vi "Get Enumerator.vi"(8 "error in (no error)":errorcluster caption="错误输入（无错误）", 11 "ArrayListClass 输入":refnum<class "ArrayListClass.lvclass"> caption="DNL_LabVIEW Object in") -> (0 "error out":errorcluster caption="错误输出", 2 "Enumerator 输出":refnum<class "Enumerator.lvclass">, 3 "ArrayListClass 输出":refnum<class "ArrayListClass.lvclass"> caption="DNL_LabVIEW Object out")   [LabVIEW 2012, in "ArrayListClass.lvclass"]
uses:
  ArrayListClass.lvclass
  Enumerator/Enumerator.lvclass
  ArrayListClass.lvclass/ArrayListClass.ctl
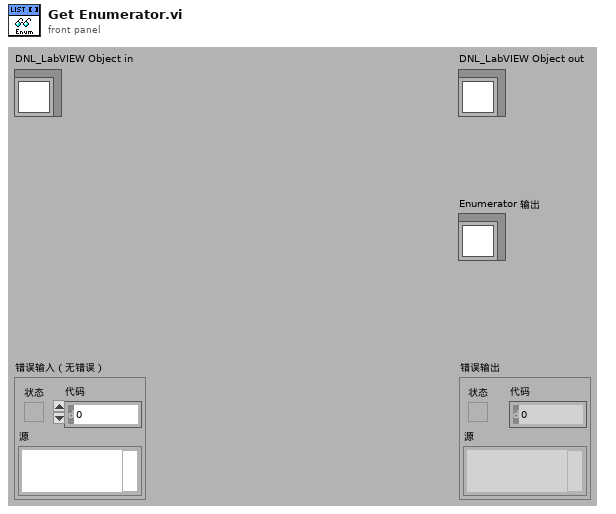
[diagram p1: front panel]
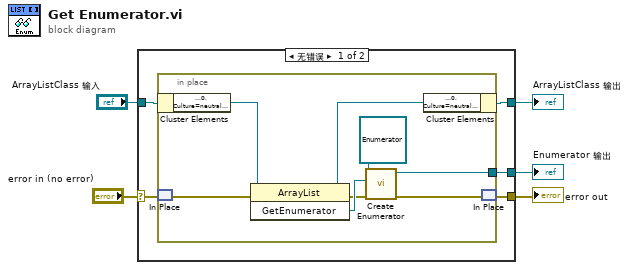
[diagram p0: block diagram]
diagram:
  n1 = case shown="无错误" "error in (no error)" {
    selector: "error in (no error)" -> [w9 w20]
    tunnel: [w6 w20] -> w4
    tunnel: [w7 w19] -> w2
    tunnel: "ArrayListClass 输入" -> [w10 w19]
    tunnel: [w8 _] -> w1
    frame No Error {
      n2 = in-place {
        in-place-border: [w11] -> w8
        n3 = in-place-cluster #1(w10) -> ("ArrayList"=w18:refnum<k24>)
        n4 = in-place-match #2(w9) -> (w17:errorcluster)
        n5 = invoke class="ArrayList" method="GetEnumerator"(reference=w18, error in=w17) -> (reference out=w13:refnum<k24>, error out=w14:errorcluster, "GetEnumerator"=w15:refnum<k24>)  [unwired: 1 in]
        n6 = call "Create Enumerator.vi"("error in (no error)"=w14, "Enumerator"=w15, "Enumerator 输入"=refnum<class "Enumerator.lvclass"> refnum ("Enumerator.lvclass")) -> ("error out"=w12:errorcluster, "Enumerator 输出"=w11:refnum<class "Enumerator.lvclass">)  [unwired: 7 in]
        n7 = in-place-cluster #1("ArrayList"=w13) -> (w7:refnum<class "ArrayListClass.lvclass">)
        n8 = in-place-match #2(w12) -> (w6:errorcluster)
      }
    }
    frame Error {
    }
  }
  "error out" <- w4
  "ArrayListClass 输出" <- w2
  "Enumerator 输出" <- w1
